vi "ProdaNG.Tree.Proc.Update.vi"(4 "Configuration":T1={"ShowUnreleased"=FALSE, "Param1"="", "ParamStartIdx"=0, "Slots"=1} {"Slots" min=1 max=2; "ParamStartIdx" min=0 max=1}, 6 "VariantFilter":string caption="Wabco Part Filter", 7 "Tree":refnum<vi>, 8 "error in (no error)":errorcluster, 11 "dbHandle in":i32) -> (0 "error out":errorcluster, 3 "dbHandle out":i32)   [LabVIEW 2016]
uses:
  ProdaNG.Configurator.Config.ctl
  ProdaNG.Configurator.Glb.vi
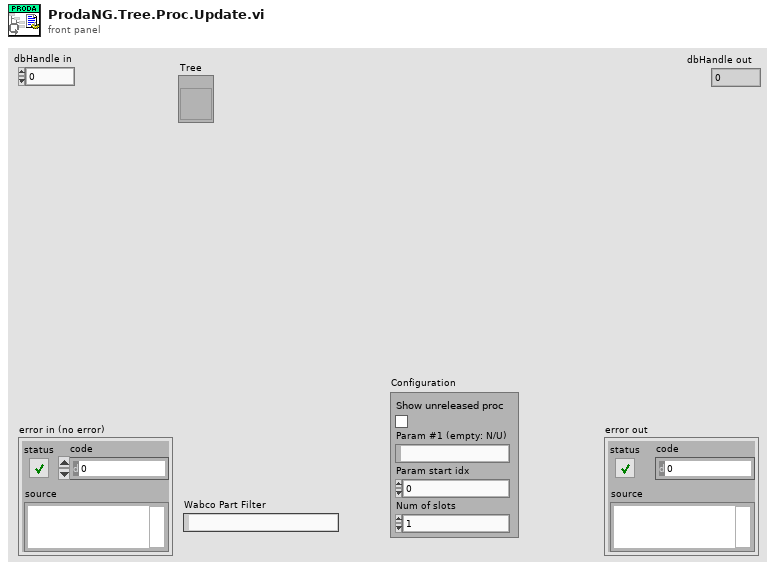
[diagram p1: front panel]
types:
  T1 = typedef "ProdaNG.Configurator.Config.ctl" = cluster{"ShowUnreleased":bool, "Param1":string, "ParamStartIdx":i32, "Slots":i32}
  T2 = cluster{"P_ID":i32, "S_ID":i32, "PS_ID":i32, "WP_ID":i32}
  T3 = typedef "ProdaNG.WabcoPart.ctl" = cluster{"i_id":i32, "workCenterId":i32, "contentId":string, "previewId":string, "mdReason":string, "mdUser":string, "mdTime":string, "productName":string, "wabcoNumber":string}
  T4 = typedef "ProdaNG.Process.ctl" = cluster{"i_id":i32, "productionLineId":i32, "releaseId":i32, "contentId":string, "previewId":string, "mdReason":string, "mdUser":string, "mdTime":string, "description":string}
  T5 = typedef "ProdaNG.ProcessStep.ctl" = cluster{"i_id":i32, "processId":i32, "systemId":i32, "releaseId":i32, "processSequence":i32, "limitYellow":dbl, "limitRed":dbl, "mdReason":string, "mdUser":string, "mdTime":string, "filename":string, "transfer":string, "description":string}
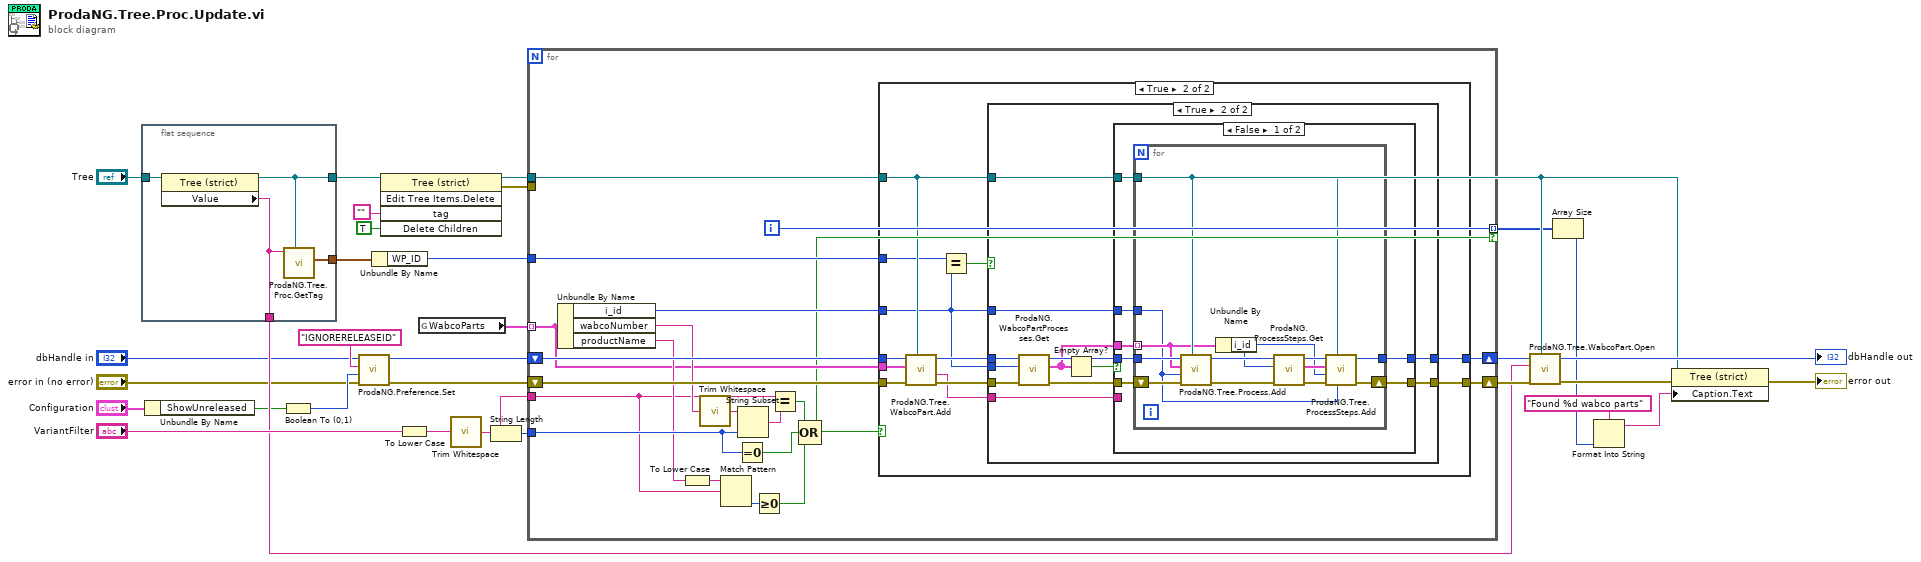
[diagram p0: block diagram]
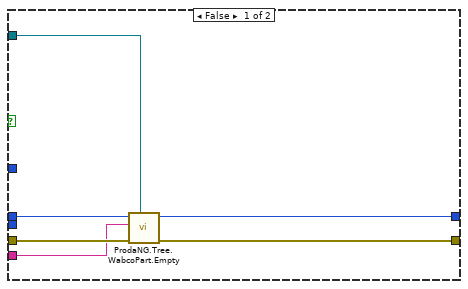
[diagram p3: hidden frame]
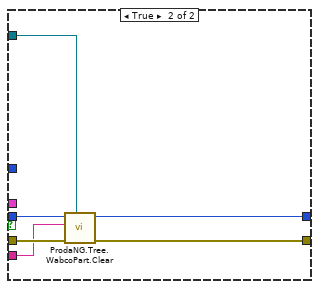
[diagram p4: hidden frame]
diagram:
  n1 = flat-sequence {
    tunnel: "Tree" -> [w34]
    tunnel: [w33] -> w24
    tunnel: [w32] -> w23
    tunnel: [w31] -> w20
    frame #0 {
      n2 = property class="Tree (strict)"(reference=w34) -> (reference out=w33:refnum<vi>, "Value"=w31:string)  [unwired: 1 in, 1 out]
      n3 = call "ProdaNG.Tree.Proc.GetTag.vi"("Tree"=w33, "Tag"=w31) -> ("Identification"=w32:T2)  [unwired: 5 in, 4 out]
    }
  }
  n4 = Unbundle By Name("Configuration") -> ("ShowUnreleased"=w1:bool)
  n5 = Boolean To (0,1)(Boolean=w1) -> (0, 1=w8:i16)
  n6 = call "ProdaNG.Preference.Set.vi"("error in"="error in (no error)", "value"=w8, "key"="IGNORERELEASEID", "dbHandleIn"="dbHandle in") -> ("error out"=w6:errorcluster, "dbHandle"=w5:i32)  [unwired: 6 in]
  n7 = Unbundle By Name(w23) -> ("WP_ID"=w22:i32)
  n8 = invoke class="Tree (strict)" method="Edit Tree Items.Delete"(reference=w24, "tag"="", "Delete Children"=TRUE ("Delete Children?")) -> (reference out=w13:refnum<vi>, error out=w26:errorcluster)  [unwired: 2 in, 3 out]
  n9 = To Lower Case(string="VariantFilter") -> (all lower case string=w17:string)
  n10 = global read "ProdaNG.Configurator.Glb.vi" "WabcoParts"() -> (w16:T3[])
  n11 = call <vilib>:"Trim Whitespace.vi"("string"=w17) -> ("trimmed string"=w18:string)  [unwired: 1 in]
  n12 = String Length(string=w18) -> (length=w19:i32)
  n13 = for {
    shift-right: [w53] -> w30
    shift-left: w5 -> [w54]
    shift-right: [w52] -> w21
    shift-left: w6 -> [w55]
    tunnel: w13 -> [w51]
    tunnel: w26 -> [_]
    tunnel: w22 -> [w50]
    tunnel: w19 -> [w45]
    tunnel: w18 -> [w38]
    tunnel: w16 -> [w37] mode=indexing
    tunnel: [w36] -> w12 mode=indexing if=w35
    i -> [w36]
    n14 = Unbundle By Name(w37) -> ("i_id"=w44:i32, "wabcoNumber"=w49:string, "productName"=w43:string)
    n15 = To Lower Case(string=w43) -> (all lower case string=w39:string)
    n16 = call <vilib>:"Trim Whitespace.vi"("string"=w49) -> ("trimmed string"=w47:string)  [unwired: 1 in]
    n17 = Match Pattern(string=w39, regular expression=w38) -> (offset past match=w41:i32)  [unwired: 1 in, 3 out]
    n18 = Equal To 0?(x=w45) -> (x = 0?=w42:bool)
    n19 = String Subset(string=w47, length (rest)=w45) -> (substring=w48:string)  [unwired: 1 in]
    n20 = Greater Or Equal To 0?(x=w41) -> (x >= 0?=w40:bool)
    n21 = Equal?(x=w38, y=w48) -> (x = y?=w46:bool)
    n22 = Compound Arithmetic op=OR(w46, w42, w40) -> (w35:bool)
    n23 = case shown="True" w35 {
      tunnel: w55 -> [w56 w65]
      tunnel: w54 -> [w57 w68]
      tunnel: [w57 w67] -> w53
      tunnel: [w56 w66] -> w52
      tunnel: w37 -> [_ w64]
      tunnel: w51 -> [_ w63]
      tunnel: w50 -> [_ w61]
      tunnel: w44 -> [_ w59]
      frame False {
      }
      frame True {
        n24 = call "ProdaNG.Tree.WabcoPart.Add.vi"("Tree"=w63, "error in (no error)"=w65, "WabcoPart"=w64) -> ("error out"=w62:errorcluster, "tag"=w58:string)  [unwired: 7 in]
        n25 = Equal?(x=w61, y=w59) -> (x = y?=w60:bool)
        n26 = case shown="True" w60 {
          tunnel: w68 -> [w73 w85]
          tunnel: [w73 w81] -> w67
          tunnel: [w70 w80] -> w66
          tunnel: w63 -> [w72 w78]
          tunnel: w62 -> [w71 w77]
          tunnel: w59 -> [_ w76]
          tunnel: w59 -> [_ w75]
          tunnel: w58 -> [w69 w74]
          frame False {
            n27 = call "ProdaNG.Tree.WabcoPart.Empty.vi"("Tree"=w72, "error in (no error)"=w71, "Tag"=w69) -> ("error out"=w70:errorcluster)  [unwired: 8 in]
          }
          frame True {
            n28 = call "ProdaNG.WabcoPartProcesses.Get.vi"("error in (no error)"=w77, "WabcoPartId"=w76, "dbHandleIn"=w85) -> ("error out"=w83:errorcluster, "Proc"=w79:T4[], "dbHandle"=w82:i32)  [unwired: 6 in]
            n29 = Empty Array?(array=w79) -> (empty?=w84:bool)
            n30 = case shown="False" w84 {
              tunnel: w83 -> [w87 w107]
              tunnel: w82 -> [w91 w108]
              tunnel: [w90 w108] -> w81
              tunnel: [w89 w104] -> w80
              tunnel: w79 -> [w92 _]
              tunnel: w78 -> [w88 w106]
              tunnel: w75 -> [w86 _]
              tunnel: w74 -> [_ w105]
              frame False {
                n31 = for {
                  tunnel: w91 -> [w103]
                  tunnel: [w96] -> w90
                  tunnel: w92 -> [w94] mode=indexing
                  shift-right: [w97] -> w89
                  shift-left: w87 -> [w101]
                  tunnel: w88 -> [w102]
                  tunnel: w86 -> [w93]
                  n32 = call "ProdaNG.Tree.Process.Add.vi"("Tree"=w102, "error in (no error)"=w101, "WabcoPartId"=w93, "ProcessStep"=w94) -> ("error out"=w100:errorcluster)  [unwired: 7 in]
                  n33 = Unbundle By Name(w94) -> ("i_id"=w95:i32)
                  n34 = call "ProdaNG.ProcessSteps.Get.vi"("error in (no error)"=w100, "processId"=w95, "dbHandleIn"=w103) -> ("error out"=w98:errorcluster, "ProcSteps"=w99:T5[], "dbHandle"=w96:i32)  [unwired: 6 in]
                  n35 = call "ProdaNG.Tree.ProcessSteps.Add.vi"("WabcoPartId"=w93, "Tree"=w102, "error in (no error)"=w98, "ProcId"=w95, "ProcSteps in"=w99) -> ("error out"=w97:errorcluster)  [unwired: 5 in, 1 out]
                }
              }
              frame True {
                n36 = call "ProdaNG.Tree.WabcoPart.Clear.vi"("Tree"=w106, "error in (no error)"=w107, "Tag"=w105) -> ("error out"=w104:errorcluster)  [unwired: 8 in]
              }
            }
          }
        }
      }
    }
  }
  "dbHandle out" <- w30
  n37 = call "ProdaNG.Tree.WabcoPart.Open.vi"("Tree"=w13, "error in (no error)"=w21, "Tag"=w20) -> ("error out"=w15:errorcluster)  [unwired: 8 in]
  n38 = Array Size(array=w12) -> (size(s)=w11:i32)
  n39 = Format Into String(format string="Found %d wabco parts", w11) -> (resulting string=w9:string)  [unwired: 2 in, 1 out]
  n40 = property class="Tree (strict)"(reference=w13, error in=w15, "Caption.Text"=w9) -> (error out=→"error out":errorcluster)  [unwired: 1 out]
